vi "spectrum_test_lx_32bit.vi"() -> ()   [LabVIEW 2017]
uses:
  <userlib>/RSA_API/RSA_API.lvlib
panel:
  out "Waveform Graph":sgl[](graph)
  in  "maxTracePoints":i32=801
  out "outTracePoints out":i32
  out "ready out":bool
  out "enable out":bool
  in  "enable":bool
  in  "refLevel":dbl=-50.0
  out "cf out":dbl
  in  "cf":dbl=2450000000.0
  out "serialNum out":string
  in  "deviceID":i32
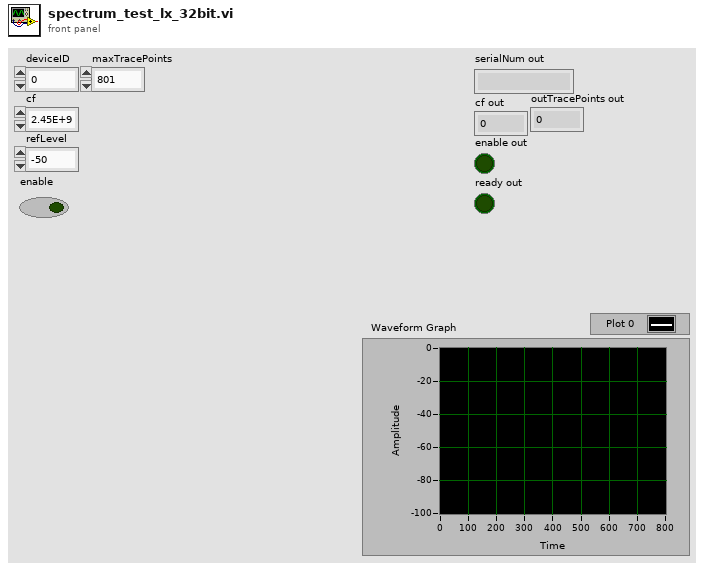
[diagram p1: front panel]
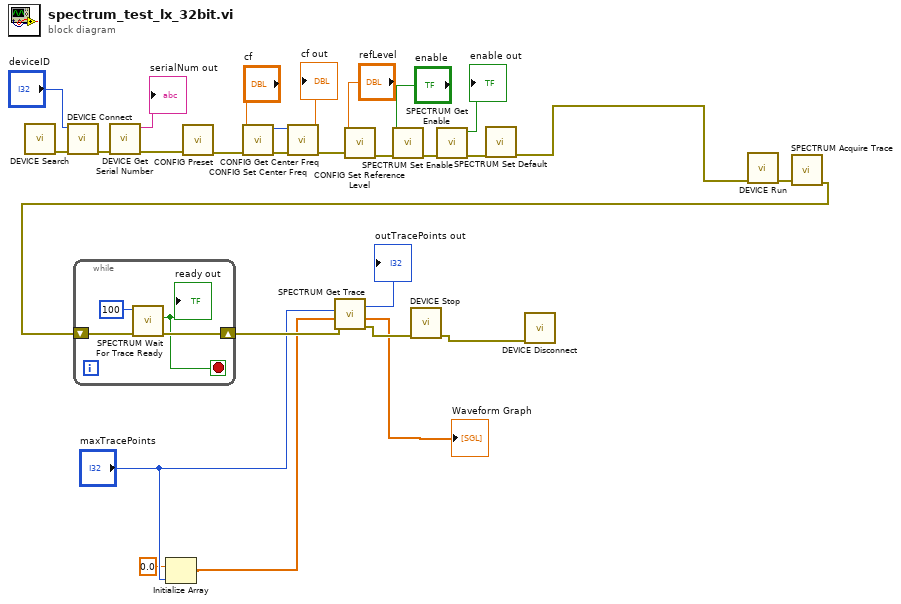
[diagram p0: block diagram]
diagram:
  n1 = call <userlib>:"DEVICE Search.vi"() -> ("error out"=w28:errorcluster)  [unwired: 10 in, 5 out]
  n2 = call <userlib>:"DEVICE Connect.vi"("error in (no error)"=w28, "deviceID"="deviceID") -> ("error out"=w26:errorcluster)  [unwired: 8 in, 1 out]
  n3 = call <userlib>:"DEVICE Get Serial Number.vi"("error in (no error)"=w26) -> ("error out"=w24:errorcluster, "serialNum out"=→"serialNum out":string)  [unwired: 8 in, 1 out]
  n4 = Initialize Array(0.0 ("element"), "maxTracePoints") -> (w5:dbl[])
  n5 = call <userlib>:"CONFIG Preset.vi"("error in (no error)"=w24) -> ("error out"=w23:errorcluster)  [unwired: 9 in, 1 out]
  n6 = call <userlib>:"CONFIG Set Center Freq.vi"("error in (no error)"=w23, "cf"="cf") -> ("error out"=w22:errorcluster, "function return"=w21:u32)  [unwired: 8 in]
  n7 = call <userlib>:"CONFIG Get Center Freq.vi"("error in (no error)"=w22, "cf"=w21) -> ("error out"=w19:errorcluster, "cf out"=→"cf out":dbl)  [unwired: 7 in, 1 out]
  n8 = call <userlib>:"CONFIG Set Reference Level.vi"("error in (no error)"=w19, "refLevel"="refLevel") -> ("error out"=w16:errorcluster)  [unwired: 8 in, 1 out]
  n9 = call <userlib>:"SPECTRUM Set Enable.vi"("error in (no error)"=w16, "enable"="enable") -> ("error out"=w15:errorcluster)  [unwired: 8 in, 1 out]
  n10 = call <userlib>:"SPECTRUM Get Enable.vi"("error in (no error)"=w15) -> ("error out"=w12:errorcluster, "enable out"=→"enable out":bool)  [unwired: 8 in, 1 out]
  n11 = call <userlib>:"SPECTRUM Set Default.vi"("error in (no error)"=w12) -> ("error out"=w1:errorcluster)  [unwired: 9 in, 1 out]
  n12 = call <userlib>:"DEVICE Run.vi"("error in (no error)"=w1) -> ("error out"=w11:errorcluster)  [unwired: 9 in, 1 out]
  n13 = call <userlib>:"SPECTRUM Acquire Trace.vi"("error in (no error)"=w11) -> ("error out"=w10:errorcluster)  [unwired: 9 in, 1 out]
  n14 = while {
    shift-right: [w31] -> w9
    shift-left: w10 -> [w32]
    stop <- w29 stop-if-true
    n15 = call <userlib>:"SPECTRUM Wait For Trace Ready.vi"("error in (no error)"=w32, "timeoutMsec"=100) -> ("error out"=w31:errorcluster, "ready out"=w29:bool)  [unwired: 7 in, 1 out]
    "ready out" <- w29
  }
  n16 = call <userlib>:"SPECTRUM Get Trace.vi"("error in (no error)"=w9, "traceData"=w5, "maxTracePoints"="maxTracePoints") -> ("error out"=w8:errorcluster, "traceData out"=→"Waveform Graph":sgl[], "outTracePoints out"=→"outTracePoints out":i32)  [unwired: 5 in, 1 out]
  n17 = call <userlib>:"DEVICE Stop.vi"("error in (no error)"=w8) -> ("error out"=w7:errorcluster)  [unwired: 9 in, 1 out]
  n18 = call <userlib>:"DEVICE Disconnect.vi"("error in (no error)"=w7) -> ()  [unwired: 9 in, 2 out]
